vi "Generate volume image path.vi"(4 "Channel to process":enum16{"Red", "Green"}(ring), 6 "Volume index":i32, 9 "Number of planes":i32, 10 "Plane index (within its volume)":i32, 11 "Folder path":path) -> (1 "Page":u32, 3 "File path":path)   [LabVIEW 2017]
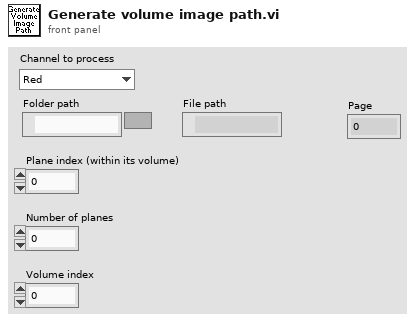
[diagram p1: front panel]
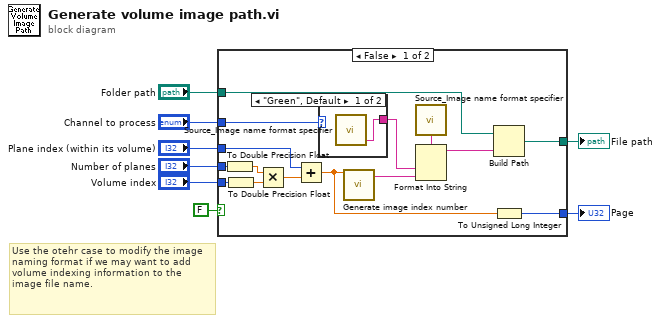
[diagram p0: block diagram]
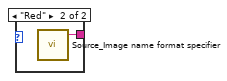
[diagram p2: hidden frame]
diagram:
  # "Use the otehr case to modify the image naming format if we may want to add volume indexing information to the image file name."
  n1 = case shown="False" FALSE {
    tunnel: "Plane index (within its volume)" -> [w23 _]
    tunnel: "Number of planes" -> [w21 _]
    tunnel: "Volume index" -> [w20 _]
    tunnel: [w19 w26] -> w5
    tunnel: "Folder path" -> [w18 w26]
    tunnel: "Channel to process" -> [w13 _]
    tunnel: [w9 _] -> w1
    frame False {
      n2 = To Double Precision Float(number=w21) -> (double precision float=w12:dbl)
      n3 = To Double Precision Float(number=w20) -> (double precision float=w11:dbl)
      n4 = Multiply(x=w12, y=w11) -> (x*y=w22:dbl)
      n5 = Add(x=w23, y=w22) -> (x+y=w10:dbl)
      n6 = case shown="\"Green\", Default" w13 {
        tunnel: [w24 w25] -> w15
        frame "Green", Default {
          n7 = call "Source_Image name format specifier.vi"() -> ("Green channel name"=w24:string)  [unwired: 5 in, 2 out]
        }
        frame "Red" {
          n8 = call "Source_Image name format specifier.vi"() -> ("Red channel name"=w25:string)  [unwired: 5 in, 2 out]
        }
      }
      n9 = call "Generate image index number.vi"("FOR loop iteration or existing number of files"=w10) -> ("Number in string representation (padded with zeroes)"=w14:string)  [unwired: 10 in]
      n10 = call "Source_Image name format specifier.vi"() -> ("Z-Stack Image name format specifier"=w16:string)  [unwired: 5 in, 2 out]
      n11 = Format Into String(format string=w16, w15, w14) -> (resulting string=w17:string)  [unwired: 2 in, 1 out]
      n12 = Build Path(base path=w18, name or relative path=w17) -> (appended path=w19:path)
      n13 = To Unsigned Long Integer(number=w10) -> (unsigned 32bit integer=w9:u32)
    }
    frame True {
    }
  }
  "File path" <- w5
  "Page" <- w1
